vi "for tests.vi"() -> ()   [LabVIEW 2020]
panel:
  out "x*y 4":dbl[](array[numeric])
  out "x*y 3":dbl[](array[numeric])
  out "Lsin":dbl[](array[numeric])
  out "Lcos":dbl[](array[numeric])
  in  "theta":dbl[](array[numeric])
  in  "L":dbl[](array[numeric])
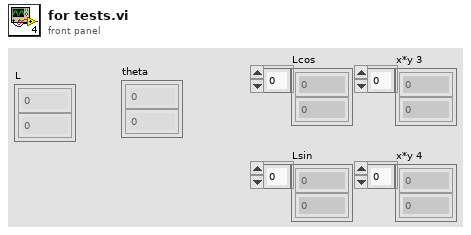
[diagram p1: front panel]
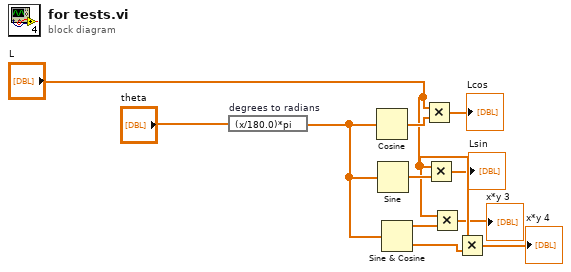
[diagram p0: block diagram]
diagram:
  n1 = expression code="(x/180.0)*pi" "degrees to radians"("theta") -> (w7:dbl[])
  n2 = Cosine(x=w7) -> (cos(x)=w10:dbl[])
  n3 = Sine(x=w7) -> (sin(x)=w8:dbl[])
  n4 = Sine & Cosine(0:w7) -> (1:w6:dbl[], 2:w5:dbl[])
  n5 = Multiply(x="L", y=w10) -> (x*y=→"Lcos":dbl[])
  n6 = Multiply(x="L", y=w8) -> (x*y=→"Lsin":dbl[])
  n7 = Multiply(x="L", y=w6) -> (x*y=→"x*y 3":dbl[])
  n8 = Multiply(x="L", y=w5) -> (x*y=→"x*y 4":dbl[])
